vi "Memory.Pointer.Clear.vi"(8 "error in (no error)":errorcluster, 11 "Pointer in":refnum<class "Memory.Pointer.Void.lvclass">) -> (0 "error out":errorcluster, 3 "Pointer out":refnum<class "Memory.Pointer.Void.lvclass">)   [LabVIEW 2016, in "LabVIEW Memory Manager.lvlib" / "Memory.Pointer.Void.lvclass"]
uses:
  Memory.Pointer.Void.lvclass
  Memory.Pointer.Void.lvclass/Memory.Pointer.Void.ctl
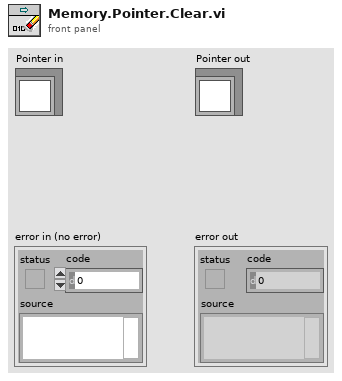
[diagram p1: front panel]
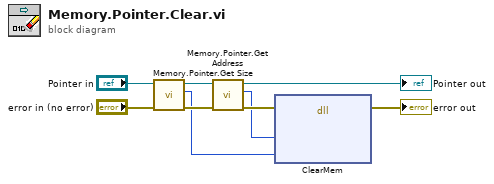
[diagram p0: block diagram]
diagram:
  n1 = call "Memory.Pointer.Get Size.vi"("error in (no error)"="error in (no error)", "Pointer in"="Pointer in") -> ("error out"=w6:errorcluster, "size"=w2:u64, "Pointer out"=w7:refnum<class "Memory.Pointer.Void.lvclass">)  [unwired: 7 in]
  n2 = call "Memory.Pointer.Get Address.vi"("error in (no error)"=w6, "Pointer in"=w7) -> ("error out"=w4:errorcluster, "address"=w1:u64, "Pointer out"=→"Pointer out":refnum<class "Memory.Pointer.Void.lvclass">)  [unwired: 7 in]
  n3 = dll-call lib="LabVIEW" fn="ClearMem"(error in=w4, "pointer"=w1, "size"=w2) -> (error out=→"error out":errorcluster)  [unwired: 5 in, 1 out]
